vi "Send Tags.vi"(8 "error in (no error)":errorcluster, 11 "Logger in.lvclass":refnum<class "Logger.lvclass">) -> (0 "error out":errorcluster, 3 "Logger out.lvclass":refnum<class "Logger.lvclass">)   [LabVIEW 2017, in "Logger.lvclass"]
uses:
  Logger.lvclass
  Logger.lvclass/Logger.ctl
  <vilib>/Skyline/Tag/Shared/typedefs/Tag Cluster Wrapper.ctl
  <vilib>/Skyline/Configuration/Configuration_class/NI Skyline Configuration.lvclass
  <vilib>/Skyline/Tag/Shared/typedefs/Tag Cluster.ctl
  <vilib>/Skyline/Tag/Shared/typedefs/DataType.ctl
  <vilib>/Skyline/Tag/Wrapper/Wrapper_class/NI Skyline Tag.lvclass
  <vilib>/Skyline/Tag/Shared/NI Skyline Tag.lvlib
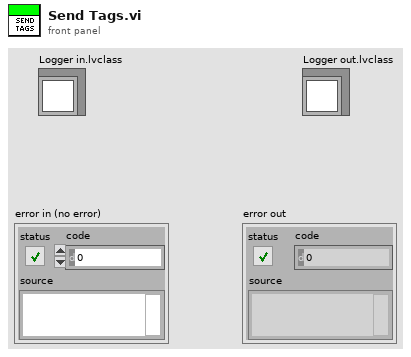
[diagram p1: front panel]
types:
  T1 = typedef "NI Skyline Tag.lvlib/Tag Cluster Wrapper.ctl" = cluster{"Configuration":refnum<class "NI Skyline Configuration.lvclass">, "Tag Cluster":T2}
  T2 = typedef "NI Skyline Tag.lvlib/Tag Cluster.ctl" = cluster{"Path":string, "Data Type":T3, "Value":variant, "Time Stamp":timestamp}
  T3 = typedef "NI Skyline Tag.lvlib/DataType.ctl" = enum32{"Double", "Integer", "String"}
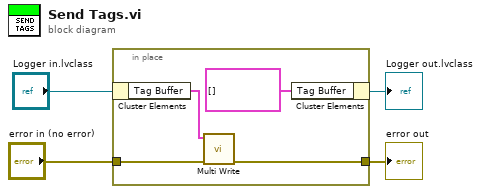
[diagram p0: block diagram]
diagram:
  n1 = in-place {
    in-place-border: "error in (no error)" -> [w8]
    in-place-border: [w7] -> w1
    n2 = in-place-cluster #1("Logger in.lvclass") -> ("Tag Buffer"=w6:T1[])
    n3 = call <vilib>:"Multi Write.vi"("error in (no error)"=w8, "tag clusters"=w6) -> ("error out"=w7:errorcluster)  [unwired: 9 in]
    n4 = in-place-cluster #1("Tag Buffer"=T1[] []) -> (→"Logger out.lvclass":refnum<class "Logger.lvclass">)
  }
  "error out" <- w1
